vi "Replace Aliases in Formula.vi"(11 "Definition in":string) -> (3 "Expanded Definition out":string)   [LabVIEW 2021, in "Formula.lvlib"]
uses:
  Formula.lvlib
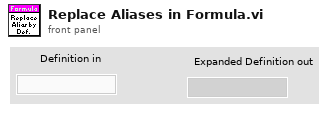
[diagram p1: front panel]
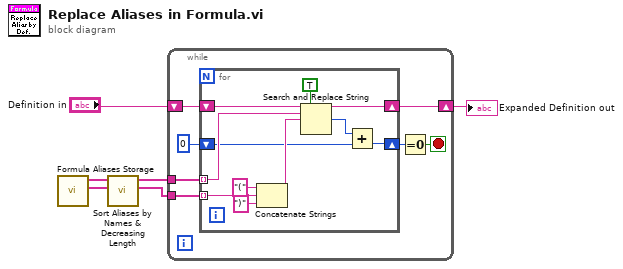
[diagram p0: block diagram]
diagram:
  n1 = call "Formula Aliases Storage.vi"() -> ("Definitions Array"=w3:string[], "Aliases Array"=w6:string[])  [unwired: 8 in, 2 out]
  n2 = call "Sort Aliases by Names & Decreasing Length.vi"("Definitions Array"=w3, "Aliases Array"=w6) -> ("Co-sorted Definitions Array"=w2:string[], "Sorted Aliases Array"=w1:string[])  [unwired: 8 in]
  n3 = while {
    tunnel: w1 -> [w13]
    tunnel: w2 -> [w12]
    shift-right: [w10] -> w4
    shift-left: "Definition in" -> [w11]
    stop <- w7 stop-if-true
    n4 = for {
      tunnel: w13 -> [w21] mode=indexing
      tunnel: w12 -> [w20] mode=indexing
      shift-right: [w23] -> w10
      shift-left: w11 -> [w24]
      shift-right: [w14] -> w8
      shift-left: 0 -> [w16]
      n5 = Concatenate Strings("(" ("string"), w20, ")" ("string")) -> (w19:string)
      n6 = Search and Replace String(replace all?=TRUE ("replace all? (F)"), input string=w24, search string=w21, replace string=w19) -> (result string=w23:string, number of replacements=w15:i32)  [unwired: 4 in, 2 out]
      n7 = Add(x=w15, y=w16) -> (x+y=w14:i32)
    }
    n8 = Equal To 0?(x=w8) -> (x = 0?=w7:bool)
  }
  "Expanded Definition out" <- w4
